vi "GetForLoopReference.vi"(8 "error in":errorcluster, 11 "ForLoop in":refnum<class "ForLoop.lvclass">) -> (0 "error out":errorcluster, 1 "reference out":refnum<vi>, 3 "ForLoop out":refnum<class "ForLoop.lvclass">)   [LabVIEW 2014, in "Raspberry Pi Compatible Compiler for LabVIEW.lvlib" / "ForLoop.lvclass"]
uses:
  ForLoop.lvclass
  Generic/Generic.lvclass
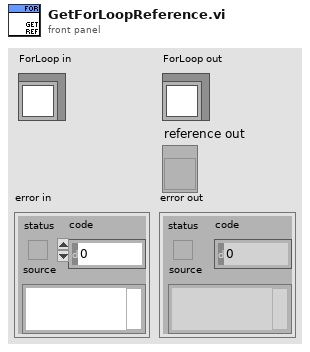
[diagram p1: front panel]
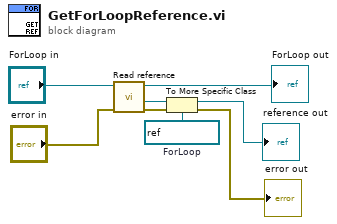
[diagram p0: block diagram]
diagram:
  w6 = refnum<vi> refnum  # ForLoop
  n1 = call "Read reference.vi"("error in"="error in", "GObject in"="ForLoop in") -> ("error out"=w7:errorcluster, "reference"=w8:refnum<vi>, "GObject out"=→"ForLoop out":refnum<class "ForLoop.lvclass">)  [unwired: 5 in]
  n2 = To More Specific Class(target class=w6, reference=w8, error in=w7) -> (specific class reference=→"reference out":refnum<vi>, error out=→"error out":errorcluster)
